vi "Prompt for Step--Init UI.vi"(8 "error in (no error)":errorcluster, 10 "Control Ref Map":map{string, refnum<vi>}(c390), 11 "Image Assertion in":refnum<class "Image Assertion.lvclass">) -> (0 "error out":errorcluster, 3 "Image Assertion out":refnum<class "Image Assertion.lvclass">)   [LabVIEW 2020, in "MacroAssert.lvlib" / "Image Assertion.lvclass"]
doc: "Initializes the user interface within the \"Prompt for Step\" VI."
uses:
  Image Assertion.lvclass
  Assertion Step/Assertion Step.lvclass
  Image Assertion.lvclass/Image Assertion.ctl
  MacroAssert.lvlib
  Support/Get Control Reference by Label (1D STR).vi
  5e651ac1-9ee7-4182-af75-eefab3161e86.vi
  6daf07e2-7199-4bc8-9aff-b1b0419c93f0.vi
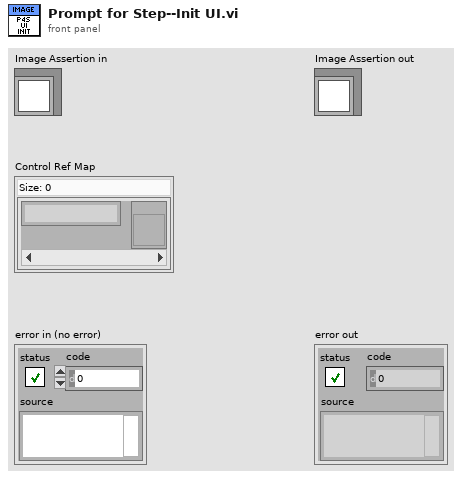
[diagram p1: front panel]
types:
  T1 = typedef "MacroAssert.lvlib/Image Assertion.lvclass/Image Assertion Type.ctl" = enum16{"Control Image", "VI Image", "Window Image"}
  T2 = typedef "MacroAssert.lvlib/Image Assertion.lvclass/Image Comparator.ctl" = enum16{"Equals", "Does not equal"}
  T3 = typedef "imagedata.ctl" = cluster{"image type":i32, "image depth":i32, "image":u8[], "mask":u8[], "colors":u32[], "Rectangle":cluster{"left":i16, "top":i16, "right":i16, "bottom":i16}}
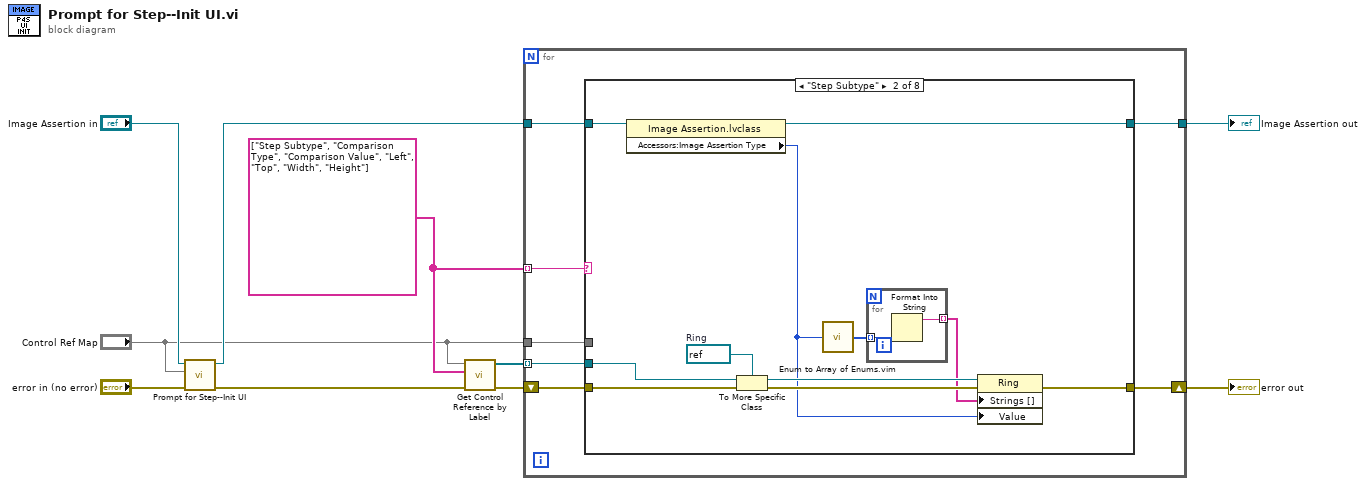
[diagram p0: block diagram]
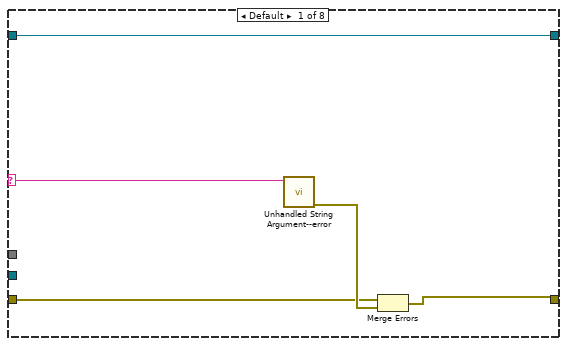
[diagram p2: hidden frame]
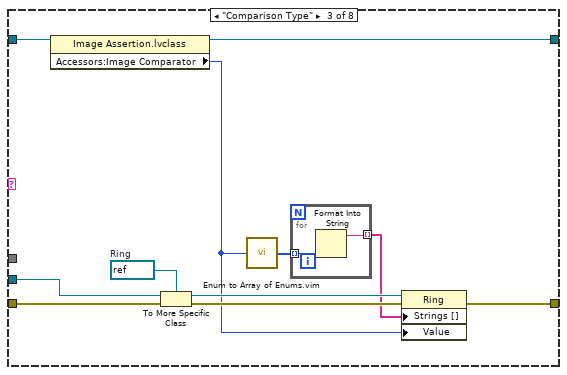
[diagram p3: hidden frame]
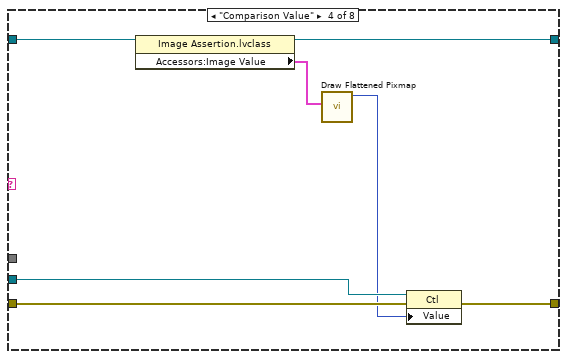
[diagram p4: hidden frame]
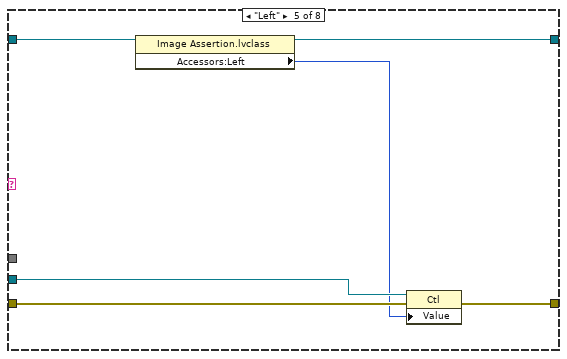
[diagram p5: hidden frame]
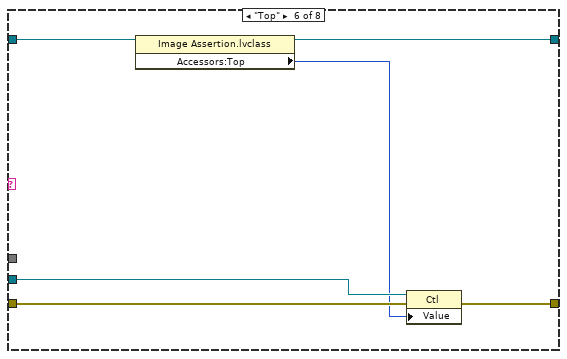
[diagram p6: hidden frame]
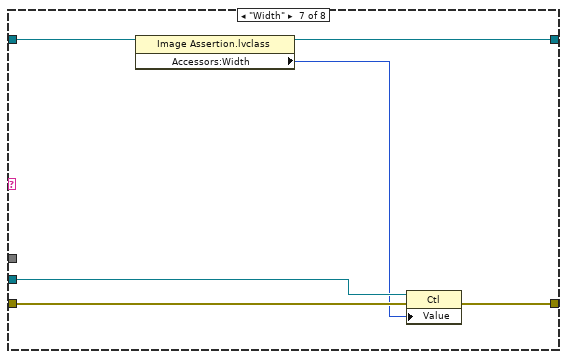
[diagram p7: hidden frame]
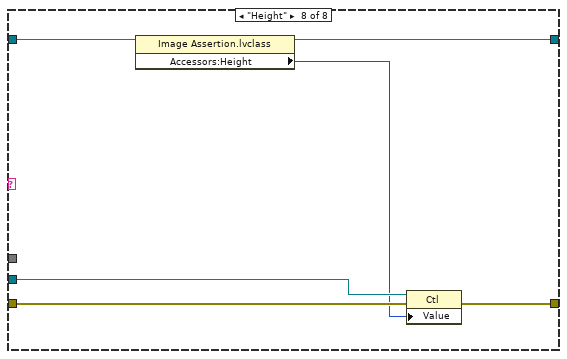
[diagram p8: hidden frame]
diagram:
  w9 = string[] ["Step Subtype", "Comparison Type", "Comparison Value", "Left", "Top", "Width", "Height"]
  n1 = call-parent "Prompt for Step--Init UI.vi"("error in (no error)"="error in (no error)", "Control Ref Map"="Control Ref Map", "Assertion Step in"="Image Assertion in") -> ("error out"=w4:errorcluster, "Assertion Step out"=w2:refnum<class "Image Assertion.lvclass">)  [unwired: 7 in]
  n2 = call-poly "Get Control Reference by Label.vi"("error in (no error)"=w4, "Control Names"=w9, "Control Ref Map"="Control Ref Map") -> ("error out"=w10:errorcluster, "Control Refs"=w8:refnum<vi>[])  [unwired: 6 in, 1 out]
  n3 = for {
    tunnel: w2 -> [w15]
    tunnel: [w13] -> w5
    tunnel: w9 -> [w16] mode=indexing
    tunnel: w8 -> [w14] mode=indexing
    shift-right: [w12] -> w7
    shift-left: w10 -> [w17]
    tunnel: "Control Ref Map" -> [w11]
    n4 = case shown="\"Step Subtype\"" w16 {
      selector: w16 -> [w18 _ _ _ _ _ _ _]
      tunnel: w17 -> [w21 w31 w44 w52 w58 w64 w70 w76]
      tunnel: w15 -> [w19 w33 w46 w55 w61 w67 w73 w79]
      tunnel: w14 -> [_ w26 w39 w53 w59 w65 w71 w77]
      tunnel: [w19 w32 w45 w54 w60 w66 w72 w78] -> w13
      tunnel: [w20 w30 w43 w51 w56 w62 w68 w74] -> w12
      tunnel: w11 -> [_ _ _ _ _ _ _ _]
      frame Default {
        n5 = call "Unhandled String Argument--error.vi"("Argument"=w18) -> ("error out"=w22:errorcluster)  [unwired: 10 in]
        n6 = Merge Errors(w21, w22) -> (w20:errorcluster)
      }
      frame "Step Subtype" {
        w27 = refnum<vi> refnum  # Ring
        n7 = property class="Image Assertion.lvclass"(reference=w33) -> (reference out=w32:refnum<class "Image Assertion.lvclass">, "Accessors:Image Assertion Type"=w24:T1)  [unwired: 1 in, 1 out]
        n8 = To More Specific Class(target class=w27, reference=w26, error in=w31) -> (specific class reference=w25:refnum<vi>, error out=w28:errorcluster)
        n9 = call "Enum to Array of Enums.vim"("enum"=w24) -> ("array of enums"=w29:T1[])
        n10 = for {
          tunnel: w29 -> [w35] mode=indexing
          tunnel: [w34] -> w23 mode=indexing
          n11 = Format Into String(w35) -> (resulting string=w34:string)  [unwired: 3 in, 1 out]
        }
        n12 = property class="Ring"(reference=w25, error in=w28, "Strings []"=w23, "Value"=w24) -> (error out=w30:errorcluster)  [unwired: 1 out]
      }
      frame "Comparison Type" {
        w40 = refnum<vi> refnum  # Ring
        n13 = property class="Image Assertion.lvclass"(reference=w46) -> (reference out=w45:refnum<class "Image Assertion.lvclass">, "Accessors:Image Comparator"=w37:T2)  [unwired: 1 in, 1 out]
        n14 = To More Specific Class(target class=w40, reference=w39, error in=w44) -> (specific class reference=w38:refnum<vi>, error out=w41:errorcluster)
        n15 = call "Enum to Array of Enums.vim"("enum"=w37) -> ("array of enums"=w42:T2[])
        n16 = for {
          tunnel: w42 -> [w48] mode=indexing
          tunnel: [w47] -> w36 mode=indexing
          n17 = Format Into String(w48) -> (resulting string=w47:string)  [unwired: 3 in, 1 out]
        }
        n18 = property class="Ring"(reference=w38, error in=w41, "Strings []"=w36, "Value"=w37) -> (error out=w43:errorcluster)  [unwired: 1 out]
      }
      frame "Comparison Value" {
        n19 = property class="Image Assertion.lvclass"(reference=w55) -> (reference out=w54:refnum<class "Image Assertion.lvclass">, "Accessors:Image Value"=w50:T3)  [unwired: 1 in, 1 out]
        n20 = call <vilib>:"Draw Flattened Pixmap.vi"("image data"=w50) -> ("new picture"=w49:picture)  [unwired: 8 in]
        n21 = property class="Ctl"(reference=w53, error in=w52, "Value"=w49) -> (error out=w51:errorcluster)  [unwired: 1 out]
      }
      frame "Left" {
        n22 = property class="Image Assertion.lvclass"(reference=w61) -> (reference out=w60:refnum<class "Image Assertion.lvclass">, "Accessors:Left"=w57:i16)  [unwired: 1 in, 1 out]
        n23 = property class="Ctl"(reference=w59, error in=w58, "Value"=w57) -> (error out=w56:errorcluster)  [unwired: 1 out]
      }
      frame "Top" {
        n24 = property class="Image Assertion.lvclass"(reference=w67) -> (reference out=w66:refnum<class "Image Assertion.lvclass">, "Accessors:Top"=w63:i16)  [unwired: 1 in, 1 out]
        n25 = property class="Ctl"(reference=w65, error in=w64, "Value"=w63) -> (error out=w62:errorcluster)  [unwired: 1 out]
      }
      frame "Width" {
        n26 = property class="Image Assertion.lvclass"(reference=w73) -> (reference out=w72:refnum<class "Image Assertion.lvclass">, "Accessors:Width"=w69:i16)  [unwired: 1 in, 1 out]
        n27 = property class="Ctl"(reference=w71, error in=w70, "Value"=w69) -> (error out=w68:errorcluster)  [unwired: 1 out]
      }
      frame "Height" {
        n28 = property class="Image Assertion.lvclass"(reference=w79) -> (reference out=w78:refnum<class "Image Assertion.lvclass">, "Accessors:Height"=w75:i16)  [unwired: 1 in, 1 out]
        n29 = property class="Ctl"(reference=w77, error in=w76, "Value"=w75) -> (error out=w74:errorcluster)  [unwired: 1 out]
      }
    }
  }
  "error out" <- w7
  "Image Assertion out" <- w5
